vi "Handshake Result.vi"(8 "error in (no error)":errorcluster, 10 "Result":T1, 11 "Listener Notifier":T3) -> (0 "error out":errorcluster)   [LabVIEW 2020, in "Stream-TCP.lvlib" / "TCP Client.lvclass"]
uses:
  TCP Client.lvclass
  Listener Notifier.ctl
  Listener Result.ctl
  Listener Status.ctl
  Stream-TCP.lvlib
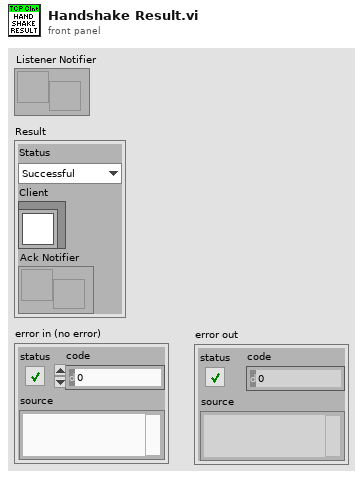
[diagram p1: front panel]
types:
  T1 = typedef "Stream-TCP.lvlib/Listener Result.ctl" = cluster{"Status":T2, "Client":refnum<class "TCP Client.lvclass">, "Ack Notifier":refnum<notifier>}
  T2 = typedef "Stream-TCP.lvlib/Listener Status.ctl" = enum16{"Successful", "Unsuccessful"}
  T3 = typedef "Stream-TCP.lvlib/Listener Notifier.ctl" = refnum<notifier>
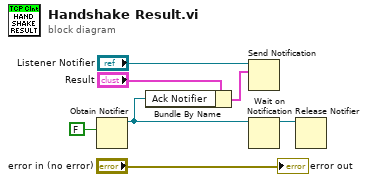
[diagram p0: block diagram]
diagram:
  n1 = Obtain Notifier(notification data type=FALSE) -> (notifier out=w3:refnum<notifier>)  [unwired: 3 in, 2 out]
  n2 = Bundle By Name(cluster="Result", "Ack Notifier"=w3) -> (w4:T1)
  n3 = Send Notification(notification=w4, notifier="Listener Notifier") -> ()  [unwired: 1 in, 2 out]
  n4 = Wait on Notification(notifier=w3) -> (notifier out=w2:refnum<notifier>)  [unwired: 3 in, 3 out]
  n5 = Release Notifier(notifier=w2) -> ()  [unwired: 2 in, 3 out]
  "error out" <- "error in (no error)"
